vi "Write_Data_to_Excel.vi"(0 "Random Data":dbl[](array[numeric])=[1.0, 2.0, 3.0, 3.0, 2.0, 5.0], 1 "Seconds into Experiment":i32[](array[numeric])=[1, 2, 3, 3, 2, 5], 2 "Vacuum Pressure":dbl[](array[numeric])=[1.0, 2.0, 3.0, 3.0, 2.0, 5.0], 3 "error in":errorcluster, 4 "Filename":path=path "test.xlsx") -> (5 "error out":errorcluster)   [LabVIEW 2015]
uses:
  <vilib>/express/express shared/transition.llb/Dynamic To Waveform Array.vi
  <vilib>/express/express signal manip/GetorSetDDTAttributes/Set DDT Attributes/SetT0.vi
  <vilib>/express/express shared/transition.llb/Waveform Array To Dynamic.vi
  <vilib>/express/express signal manip/GetorSetDDTAttributes/Set DDT Attributes/Set DDT Properties.xnode
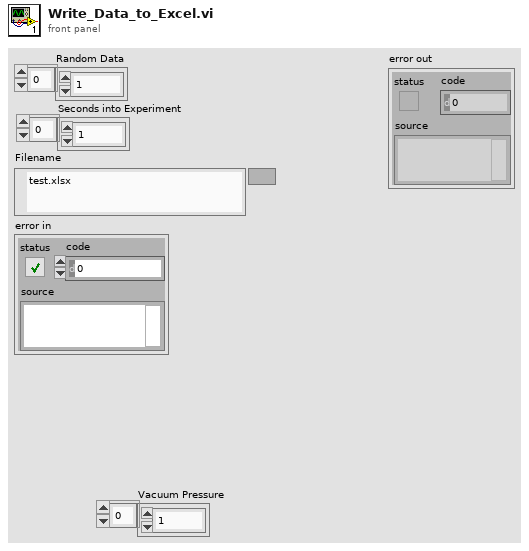
[diagram p1: front panel]
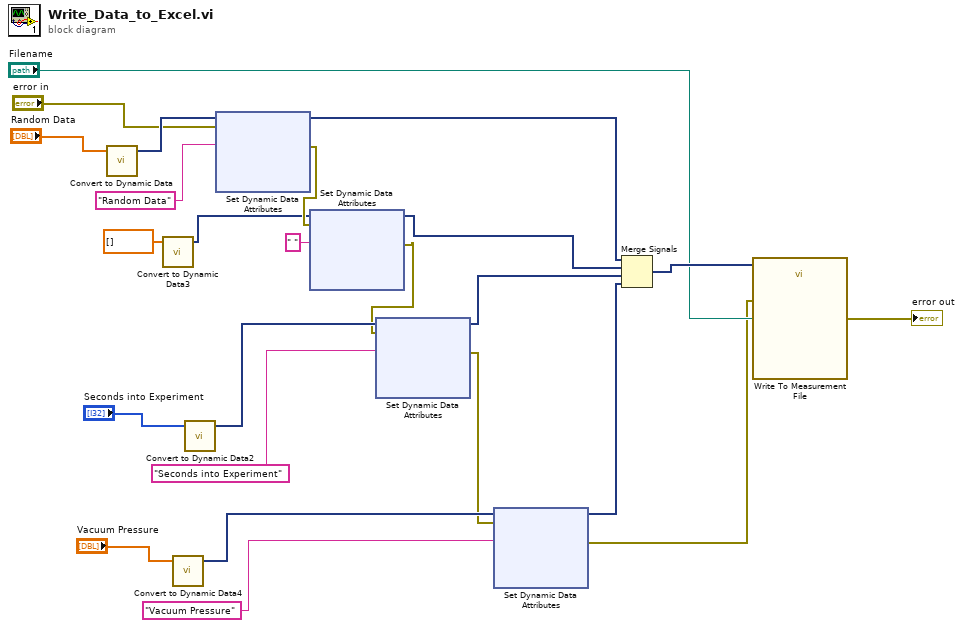
[diagram p0: block diagram]
diagram:
  n1 = call "Convert to Dynamic Data"("Array"="Random Data") -> ("Dynamic Data Type"=w20:dynamicdata)  [unwired: 3 in]
  n2 = call "Convert to Dynamic Data3"("Array"=dbl[] []) -> ("Dynamic Data Type"=w1:dynamicdata)  [unwired: 3 in]
  n3 = call "Convert to Dynamic Data4"("Array"="Vacuum Pressure") -> ("Dynamic Data Type"=w14:dynamicdata)  [unwired: 3 in]
  n4 = call "Convert to Dynamic Data2"("Array"="Seconds into Experiment") -> ("Dynamic Data Type"=w21:dynamicdata)  [unwired: 3 in]
  n5 = xnode "Set Dynamic Data Attributes"("Signals In"=w20, "error in"="error in", "Signal Name"="Random Data") -> ("Signals Out"=w17:dynamicdata, "error out"=w4:errorcluster)  [unwired: 1 in]
  n6 = xnode "Set Dynamic Data Attributes"("Signals In"=w1, "error in"=w4, "Signal Name"=" ") -> ("Signals Out"=w6:dynamicdata, "error out"=w5:errorcluster)  [unwired: 1 in]
  n7 = xnode "Set Dynamic Data Attributes"("Signals In"=w21, "error in"=w5, "Signal Name"="Seconds into Experiment") -> ("Signals Out"=w12:dynamicdata, "error out"=w9:errorcluster)  [unwired: 1 in]
  n8 = xnode "Set Dynamic Data Attributes"("Signals In"=w14, "error in"=w9, "Signal Name"="Vacuum Pressure") -> ("Signals Out"=w11:dynamicdata, "error out"=w8:errorcluster)  [unwired: 1 in]
  n9 = Merge Signals(w17, w6, w12, w11) -> (w18:dynamicdata)
  n10 = call "Write To Measurement File"("Signals"=w18, "error in (no error)"=w8, "Filename"="Filename") -> ("error out"=→"error out":errorcluster)  [unwired: 14 in, 2 out]
